vi "Errorbar1006.vi"   [LabVIEW 2013]
uses:
  <vilib>/Heliosphere Research LLC/Advanced Plotting Toolkit/api_plotting/ErrorbarProperties.ctl
  <vilib>/Heliosphere Research LLC/Advanced Plotting Toolkit/typedefs/PlotColor.ctl
  <vilib>/Heliosphere Research LLC/Advanced Plotting Toolkit/properties/Display.ctl
  <vilib>/Heliosphere Research LLC/Advanced Plotting Toolkit/Advanced Plotting Toolkit.lvlib
types:
  T1 = typedef "Advanced Plotting Toolkit.lvlib/PlotColor.ctl" = u32
  T2 = typedef "Advanced Plotting Toolkit.lvlib/ErrorbarProperties.ctl" = cluster{"Color":T1, "Line Width":dbl, "Cap Size":dbl, "Display":T3}
  T3 = typedef "Advanced Plotting Toolkit.lvlib/Display.ctl" = cluster{"Alpha":dbl, "Z Order":dbl}
  T4 = typedef "Advanced Plotting Toolkit.lvlib/PlotID.ctl" = i32
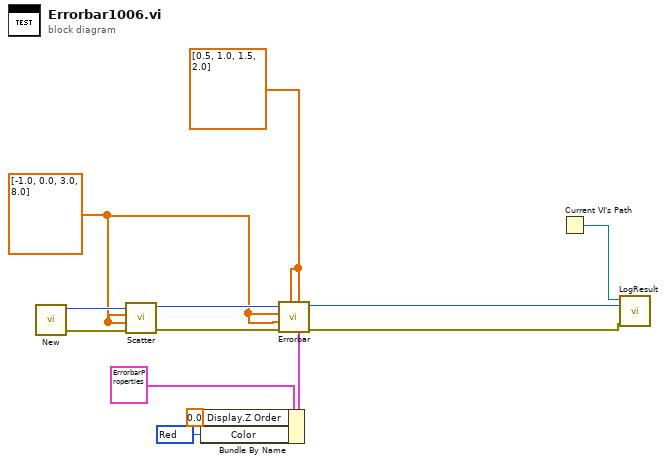
[diagram p0: block diagram]
diagram:
  w1 = T1 16711680 items=["Automatic"=2147483647, "Black"=0, "White"=16777215, "Red"=16711680, "Green"=2263842, "Blue"=255, "Cyan"=65535, "Magenta"=16711935, "Yellow"=16776960] ("Color")
  w5 = dbl[] [0.5, 1.0, 1.5, 2.0] ("X Errors")
  w6 = dbl[] [-1.0, 0.0, 3.0, 8.0] ("X Data")
  n1 = call <vilib>:"New.vi"() -> ("error out"=w7:errorcluster, "Plot ID"=w10:T4)  [unwired: 10 in]
  n2 = call <vilib>:"Scatter.vi"("error in (no error)"=w7, "Y Data"=w6, "X Data"=w6, "Plot ID"=w10) -> ("error out"=w8:errorcluster, "Plot ID Out"=w9:T4)  [unwired: 6 in]
  n3 = Bundle By Name(cluster=T2 {"Color"=2147483647, "Line Width"=nan, "Cap Size"=nan, "Display"={"Alpha"=nan, "Z Order"=nan}} ("Errorbar Properties"), "Display.Z Order"=0.0 ("Line Width"), "Color"=w1) -> (w3:T2)
  n4 = call <vilib>:"Errorbar.vi"("Properties"=w3, "Y Errors"=w5, "X Errors"=w5, "error in (no error)"=w8, "Y Data"=w6, "X Data"=w6, "Plot ID"=w9) -> ("error out"=w11:errorcluster, "Plot ID out"=w12:T4)  [unwired: 3 in]
  n5 = Current VI's Path() -> (path=w13:path)
  n6 = call "LogResult.vi"("Test Result"=w11, "Test Artifact"=w12, "VI Path"=w13) -> ()  [unwired: 9 in]
